vi "getDefaultO3Cal.vi"(7 "LWRS":refnum<class "Web Request.lvclass">) -> ()   [LabVIEW 2014]
uses:
  <vilib>/wsapi/Web Request.lvclass
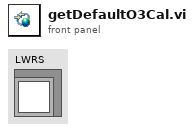
[diagram p1: front panel]
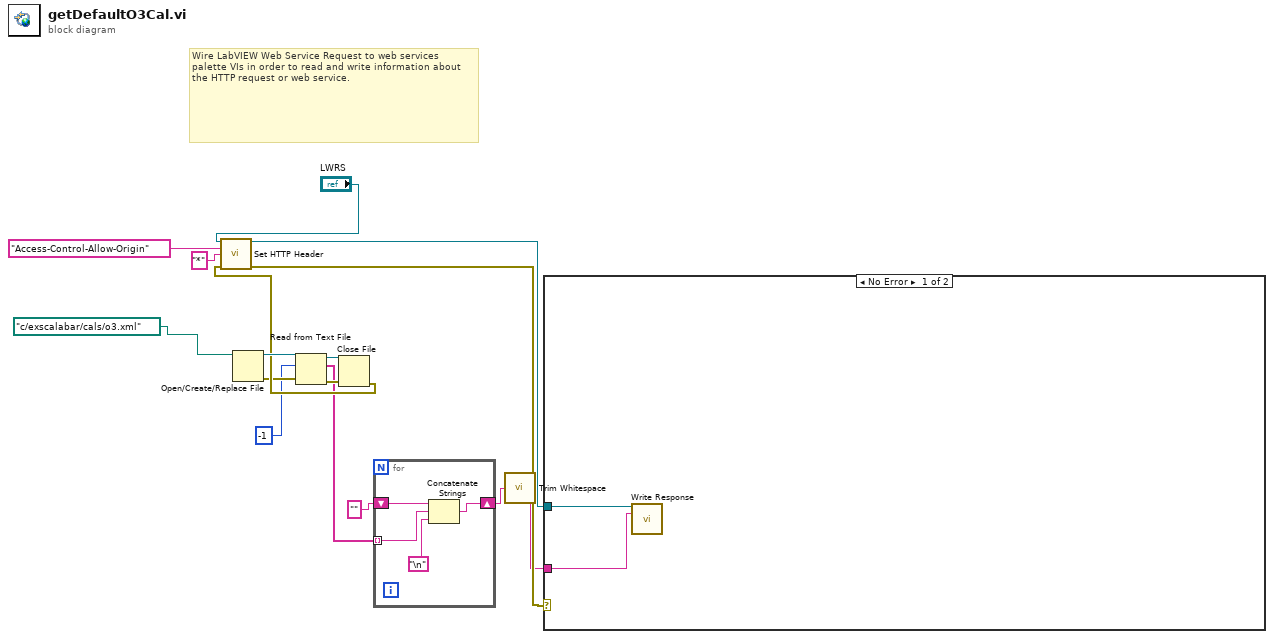
[diagram p0: block diagram]
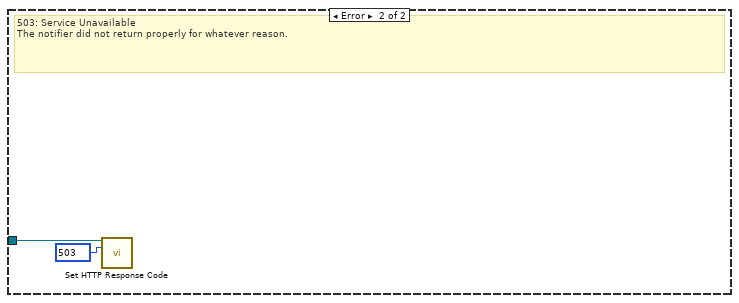
[diagram p2: hidden frame]
diagram:
  # "Wire LabVIEW Web Service Request to web services palette VIs in order to read and write information about the HTTP request or web service."
  n1 = Open/Create/Replace File(file path (use dialog)=path "c:/exscalabar/cals/o3.xml" ("Folder Path")) -> (refnum out=w10:refnum<file>, error out=w6:errorcluster)  [unwired: 5 in, 1 out]
  n2 = Read from Text File(file (use dialog)=w10, count=-1, error in=w6) -> (refnum out=w8:refnum<file>, text=w4:string[], error out=w9:errorcluster)  [unwired: 1 in, 1 out]
  n3 = Close File(refnum=w8, error in=w9) -> (error out=w7:errorcluster)  [unwired: 1 out]
  n4 = call <vilib>:"Set HTTP Header.vi"("LabVIEW Web Service Request"="LWRS", "header"="Access-Control-Allow-Origin", "header value"="*", "error in (no error)"=w7) -> ("LabVIEW Web Service Request out"=w13:refnum<class "Web Request.lvclass">, "error out"=w12:errorcluster)  [unwired: 10 in]
  n5 = for {
    tunnel: w4 -> [w20] mode=indexing
    shift-right: [w18] -> w2
    shift-left: "" -> [w19]
    n6 = Concatenate Strings(w19, w20, "\n") -> (w18:string)
  }
  n7 = call <vilib>:"Trim Whitespace.vi"("string"=w2) -> ("trimmed string"=w1:string)  [unwired: 1 in]
  n8 = case shown="No Error" w12 {
    tunnel: w13 -> [w22 w24]
    tunnel: w1 -> [w21 _]
    frame No Error {
      n9 = call <vilib>:"Write Response.vi"("LabVIEW Web Service Request"=w22, "response string"=w21) -> ()  [unwired: 12 in, 2 out]
    }
    frame Error {
      w23 = 503 items=["100"=100, "101"=101, "200"=200, "201"=201, "202"=202, "203"=203, "204"=204, "205"=205, "206"=206, "300"=300, "301"=301, "302"=302, "303"=303, "304"=304, "305"=305, "306"=306, "307"=307, "400"=400, "401"=401, "402"=402, "403"=403, "404"=404, "405"=405, "406"=406, "407"=407, "408"=408, "409"=409, "410"=410, "411"=411, "412"=412, "413"=413, "414"=414, "415"=415, "416"=416, "417"=417, "500"=500, "501"=501, "502"=502, "503"=503, "504"=504, "505"=505] ("response code (200)")
      # "503: Service Unavailable\nThe notifier did not return properly for whatever reason."
      n10 = call <vilib>:"Set HTTP Response Code.vi"("LabVIEW Web Service Request"=w24, "response code (200)"=w23) -> ()  [unwired: 12 in, 2 out]
    }
  }
